vi "Set message.vi"(10 "WampMessage MsgPack":refnum<class "WampMessage MsgPack.lvclass">, 11 "HandlePublished MsgPack in":refnum<class "HandlePublished MsgPack.lvclass">) -> (3 "HandlePublished MsgPack out":refnum<class "HandlePublished MsgPack.lvclass">)   [LabVIEW 2020, in "wamplv.lvlib" / "HandlePublished MsgPack.lvclass"]
uses:
  HandlePublished MsgPack.lvclass
  HandlePublished MsgPack.lvclass/HandlePublished MsgPack.ctl
  SerialisedMessages/MsgPackMessage/WampMessage MsgPack.lvclass
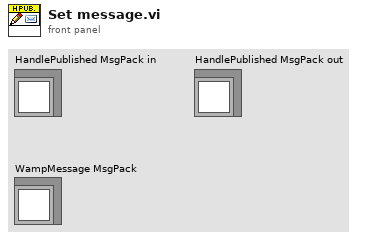
[diagram p1: front panel]
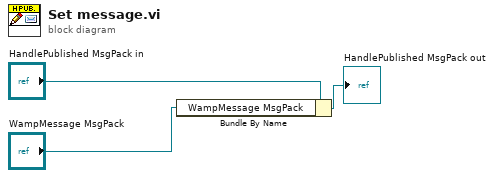
[diagram p0: block diagram]
diagram:
  n1 = Bundle By Name(cluster="HandlePublished MsgPack in", "WampMessage MsgPack"="WampMessage MsgPack") -> (→"HandlePublished MsgPack out":refnum<class "HandlePublished MsgPack.lvclass">)
